vi "PCI Configuration.Burst Interval.Get.vi"(8 "error in (no error)":errorcluster, 11 "GE 5565PIORC":refnum<class "GE 5565PIORC.lvclass">) -> (0 "error out":errorcluster, 2 "PCI Burst Interval (ns)":u8, 3 "GE 5565PIORC out":refnum<class "GE 5565PIORC.lvclass">)   [LabVIEW 2016, in "GE 5565PIORC.lvclass"]
uses:
  GE 5565PIORC.lvclass
  Controls/Registers.PCI Configuration.ctl
  GE 5565PIORC.lvclass/GE 5565PIORC.ctl
  <vilib>/Instr/_visa.llb/VISA Register Access Address Space.ctl
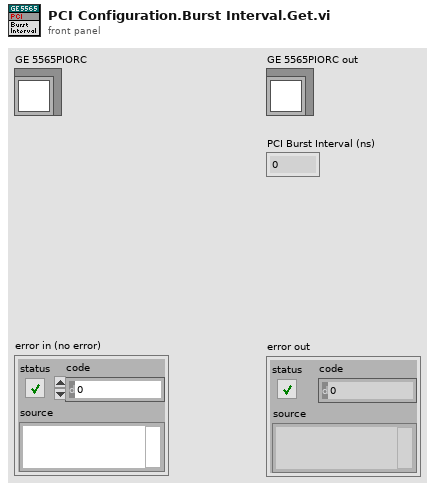
[diagram p1: front panel]
types:
  T1 = typedef "GE 5565PIORC.lvclass/Registers.PCI Configuration.ctl" = enum16{"PCI Configuration ID", "PCI Command", "PCI Status", "PCI Revision ID", "PCI Class Code", "PCI Cache Line Size", "PCI Latency Timer", "PCI Header Type", "PCI Built-In Self-Test", "PCI BAR 0", "PCI BAR 1", "PCI BAR 2", "PCI BAR 3", "PCI BAR 4", "PCI BAR 5", "PCI Cardbus CIS Pointer", "PCI Subsystem Vendor ID", "PCI Subsytem ID", "PCI Expansion ROM Base", "PCI Capability Pointer", "PCI Interrupt Line", "PCI Interrupt Pin", "PCI Min_Gnt", "PCI Max_Lat"}
  T2 = typedef "VISA Register Access Address Space.ctl" = u16
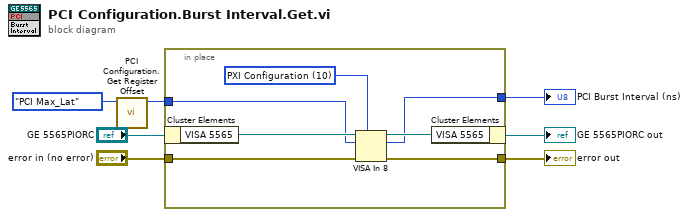
[diagram p0: block diagram]
diagram:
  n1 = call "PCI Configuration.Get Register Offset.vi"("PCI Configuration Register"=Registers.PCI_Configuration."PCI Max_Lat") -> ("Offset"=w1:u32)  [unwired: 10 in]
  n2 = in-place {
    in-place-border: "error in (no error)" -> [w12]
    in-place-border: [w11] -> w5
    in-place-border: [w9] -> w3
    in-place-border: w1 -> [w8]
    w10 = T2 10 items=["VXI/VME A16"=1, "VXI/VME A24"=2, "VXI/VME A32"=3, "VXI/VME A64"=4, "PXI Memory Allocations"=9, "PXI Configuration"=10, "PXI BAR0"=11, "PXI BAR1"=12, "PXI BAR2"=13, "PXI BAR3"=14, "PXI BAR4"=15, "PXI BAR5"=16] ("Address Space")
    n3 = in-place-cluster #1("GE 5565PIORC") -> ("VISA 5565"=w14:refnum<visa-resource-name>)
    n4 = VISA In 8(7:w10, 8:w12, 10:w8, 11:w14) -> (0:w11:errorcluster, 2:w9:u8, 3:w13:refnum<visa-resource-name>)
    n5 = in-place-cluster #1("VISA 5565"=w13) -> (→"GE 5565PIORC out":refnum<class "GE 5565PIORC.lvclass">)
  }
  "error out" <- w5
  "PCI Burst Interval (ns)" <- w3
